vi "Autonomous Independent.vi"() -> ()   [LabVIEW 2016]
doc: "This VI is called when autonomous begins, and will automatically be terminated when autonomous ends. You can carry out timed or sensor driven robot movement independently without needing to return to the caller."
uses:
  <vilib>/Rock Robotics/WPI/Utilities/WPI_GetSetVariantRefNum.vi
  <vilib>/Rock Robotics/Network Tables/NT Read String.vi
  <vilib>/Rock Robotics/Network Tables/NT Write Numeric Array.vi
  <vilib>/Rock Robotics/WPI/RobotDrive/WPI_RobotDriveArcadeDrive_Standard(NoSaturation).vi
  <vilib>/Rock Robotics/Network Tables/NT Write Number.vi
  Robot Global Data.vi
  <vilib>/Rock Robotics/WPI/Counter/WPI_CounterDigitalInputToDigitalSource.vi
  <vilib>/Rock Robotics/SystemInterfaces/DIO/FPGA_DIOChannel.ctl
panel:
  out "Hook Center Cons":dbl
  out "gyro":dbl
  out "sonar distance (inches)":dbl
  out "Encoder Loop":dbl
  out "Encoder Loop":string
  out "Current Movement, for debugging 2":T1 {"Y Joystick Value" scale=1.0..-1.0; "X Joystick Value" scale=-1.0..1.0}
  in  "Array of robot movements 2":T2(array[cluster])=[{"X Joystick Value"=0.39393939393939403, "Y Joystick Value"=0.0, "Delay (sec)"=1.0, "Movement Name"="turn"}, {"X Joystick Value"=-0.3737373737373737, "Y Joystick Value"=0.0, "Delay (sec)"=1.0, "Movement Name"="turn back"}] {"Y Joystick Value" scale=1.0..-1.0; "X Joystick Value" scale=-1.0..1.0}
  out "Current Movement, for debugging":T1 {"Y Joystick Value" scale=1.0..-1.0; "X Joystick Value" scale=-1.0..1.0}
  in  "Array of robot movements":T2(array[cluster])=[{"X Joystick Value"=0.39393939393939403, "Y Joystick Value"=0.0, "Delay (sec)"=1.0, "Movement Name"="turn"}, {"X Joystick Value"=-0.3737373737373737, "Y Joystick Value"=0.0, "Delay (sec)"=1.0, "Movement Name"="turn back"}] {"Y Joystick Value" scale=1.0..-1.0; "X Joystick Value" scale=-1.0..1.0}
  # "Sensor Readings\nConstanly updated in\nwhile loopes"
  # "Be sure to right-click and choose Data Operations>>Make Current Value default if you want to save the array values with the VI"
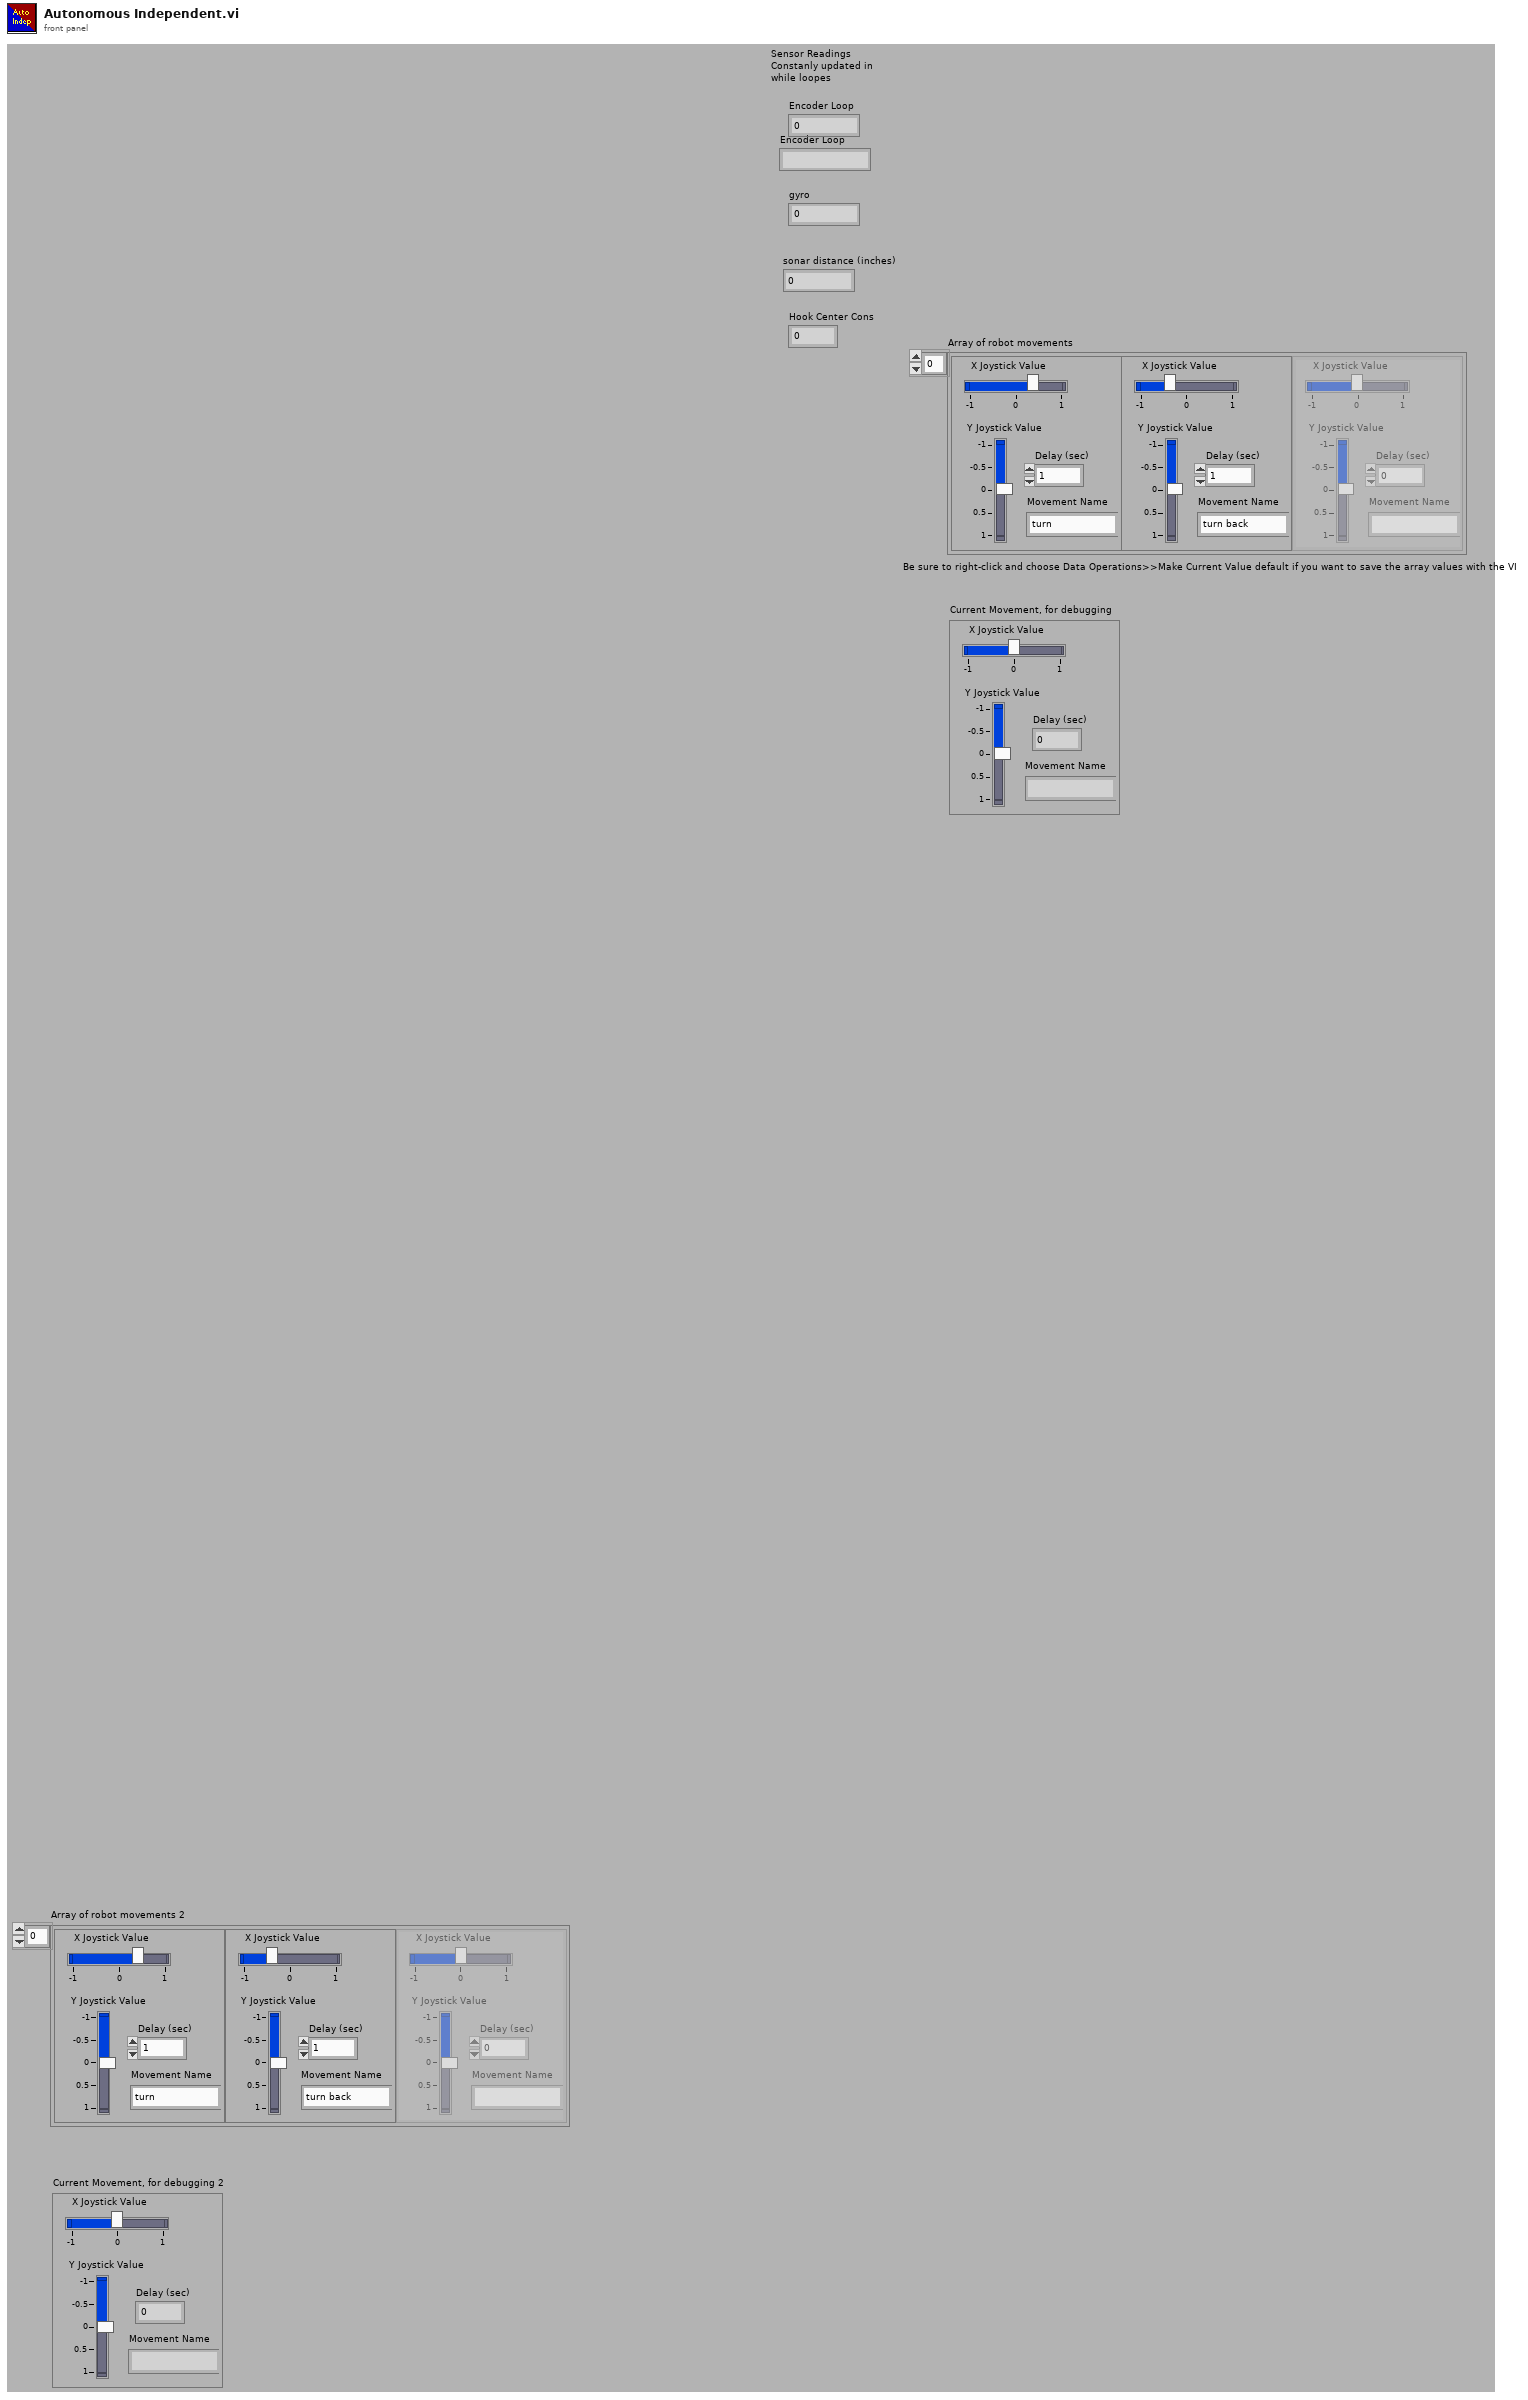
[diagram p1: front panel]
types:
  T1 = cluster{"X Joystick Value":dbl, "Y Joystick Value":dbl, "Delay (sec)":dbl, "Movement Name":string}
  T2 = cluster{"X Joystick Value":dbl, "Y Joystick Value":dbl, "Delay (sec)":dbl, "Movement Name":string}[]
  T3 = typedef "FPGA_DIOChannel.ctl" = enum8{"DIO 0", "DIO 1", "DIO 2", "DIO 3", "DIO 4", "DIO 5", "DIO 6", "DIO 7", "DIO 8", "DIO 9", "DIO MXP 0", "DIO MXP 1", "DIO MXP 2", "DIO MXP 3", "DIO MXP 4", "DIO MXP 5", "DIO MXP 6", "DIO MXP 7", "DIO MXP 8", "DIO MXP 9", "DIO MXP 10", "DIO MXP 11", "DIO MXP 12", "DIO MXP 13", "DIO MXP 14", "DIO MXP 15", "SPI Port CS1", "SPI Port CS2", "SPI Port CS3", "SPI Port MISO", "SPI Port MOSI", "Invalid"}
  T4 = typedef "WPI_DigitalInputDevRef.ctl" = cluster{"DevStatus":errorcluster, "DIO Channel":T3}
  T5 = typedef "FPGA_CounterEncoderSourceConvertionLVSourceType.ctl" = cluster{"DevStatus":errorcluster, "AnalogTriggerMode?":bool, "DigitalMode":cluster{"DIO Channel":T6}, "AnalogTriggerMode":cluster{"AnalogTriggerIndex":T7, "OutputType":T8}}
  T6 = typedef "FPGA_DIODigitalSourceChannel.ctl" = enum8{"DIO 0", "DIO 1", "DIO 2", "DIO 3", "DIO 4", "DIO 5", "DIO 6", "DIO 7", "DIO 8", "DIO 9", "DIO MXP 0", "DIO MXP 1", "DIO MXP 2", "DIO MXP 3", "DIO MXP 4", "DIO MXP 5", "DIO MXP 6", "DIO MXP 7", "DIO MXP 8", "DIO MXP 9", "DIO MXP 10", "DIO MXP 11", "DIO MXP 12", "DIO MXP 13", "DIO MXP 14", "DIO MXP 15", "Disabled"}
  T7 = typedef "FPGA_AnalogTriggerIndex.ctl" = enum8{"Trig 0", "Trig 1", "Trig 2", "Trig 3", "Trig 4", "Trig 5", "Trig 6", "Trig 7", "Invalid"}
  T8 = typedef "FPGA_AnalogTriggerOutType.ctl" = enum16{"InWindow", "TriggerState", "Rising", "Falling"}
  T9 = typedef "WPI_EncoderDevRef.ctl" = cluster{"DevStatus":errorcluster, "EncoderIndex":T10, "CounterIndex":T11, "DistancePerCount":dbl, "Decoding Type":T12}
  T10 = typedef "FPGA_EncoderIdx.ctl" = enum8{"Enc 0", "Enc 1", "Enc 2", "Enc 3", "Enc 4", "Enc 5", "Enc 6", "Enc 7", "Invalid"}
  T11 = typedef "FPGA_CounterCtrSystemIndex.ctl" = enum8{"Ctr 0", "Ctr 1", "Ctr 2", "Ctr 3", "Ctr 4", "Ctr 5", "Ctr 6", "Ctr 7", "Invalid"}
  T12 = typedef "WPI_EncoderType.ctl" = enum16{"1x", "2x", "4x"}
  T13 = typedef "WPI_JoystickDevRef.ctl" = cluster{"Device":T14}
  T14 = typedef "WPI_JoystickDeviceEnum.ctl" = enum16{"USB 0", "USB 1", "USB 2", "USB 3", "USB 4", "USB 5"}
  T15 = typedef "WPI_DriverStationPositionInfo.ctl" = enum16{"1", "2", "3"}
  T16 = typedef "WPI_RobotDriveDevRef.ctl" = cluster{"DevStatus":errorcluster, "Motors[]":T17[], "Square Inputs":bool, "Max Output":dbl}
  T17 = typedef "WPI_MotorControlDeviceRef.ctl" = cluster{"DeviceStatus":errorcluster, "Type":T18, "PWM":cluster{"PWM Channel":T19, "DeadBand":T20}, "CAN":cluster{"Device Number":u8, "SetOutput VI Ref":variant, "GetOutput VI Ref":variant, "Enable VI Ref":variant, "Disable VI Ref":variant, "Data":variant}, "Invert":bool}
  T18 = typedef "WPI_MotorControlType.ctl" = enum16{"PWM", "CAN"}
  T19 = typedef "FPGA_DIOPWMChannel.ctl" = enum8{"PWM 0", "PWM 1", "PWM 2", "PWM 3", "PWM 4", "PWM 5", "PWM 6", "PWM 7", "PWM 8", "PWM 9", "PWM MXP 0", "PWM MXP 1", "PWM MXP 2", "PWM MXP 3", "PWM MXP 4", "PWM MXP 5", "PWM MXP 6", "PWM MXP 7", "PWM MXP 8", "PWM MXP 9", "Invalid"}
  T20 = typedef "WPI_PWMDeadband.ctl" = cluster{"Name":string, "maxPositivePwm":i32, "minPositivePwm":i32, "centerPwm":i32, "maxNegativePwm":i32, "minNegativePwm":i32, "angularRange":u16}
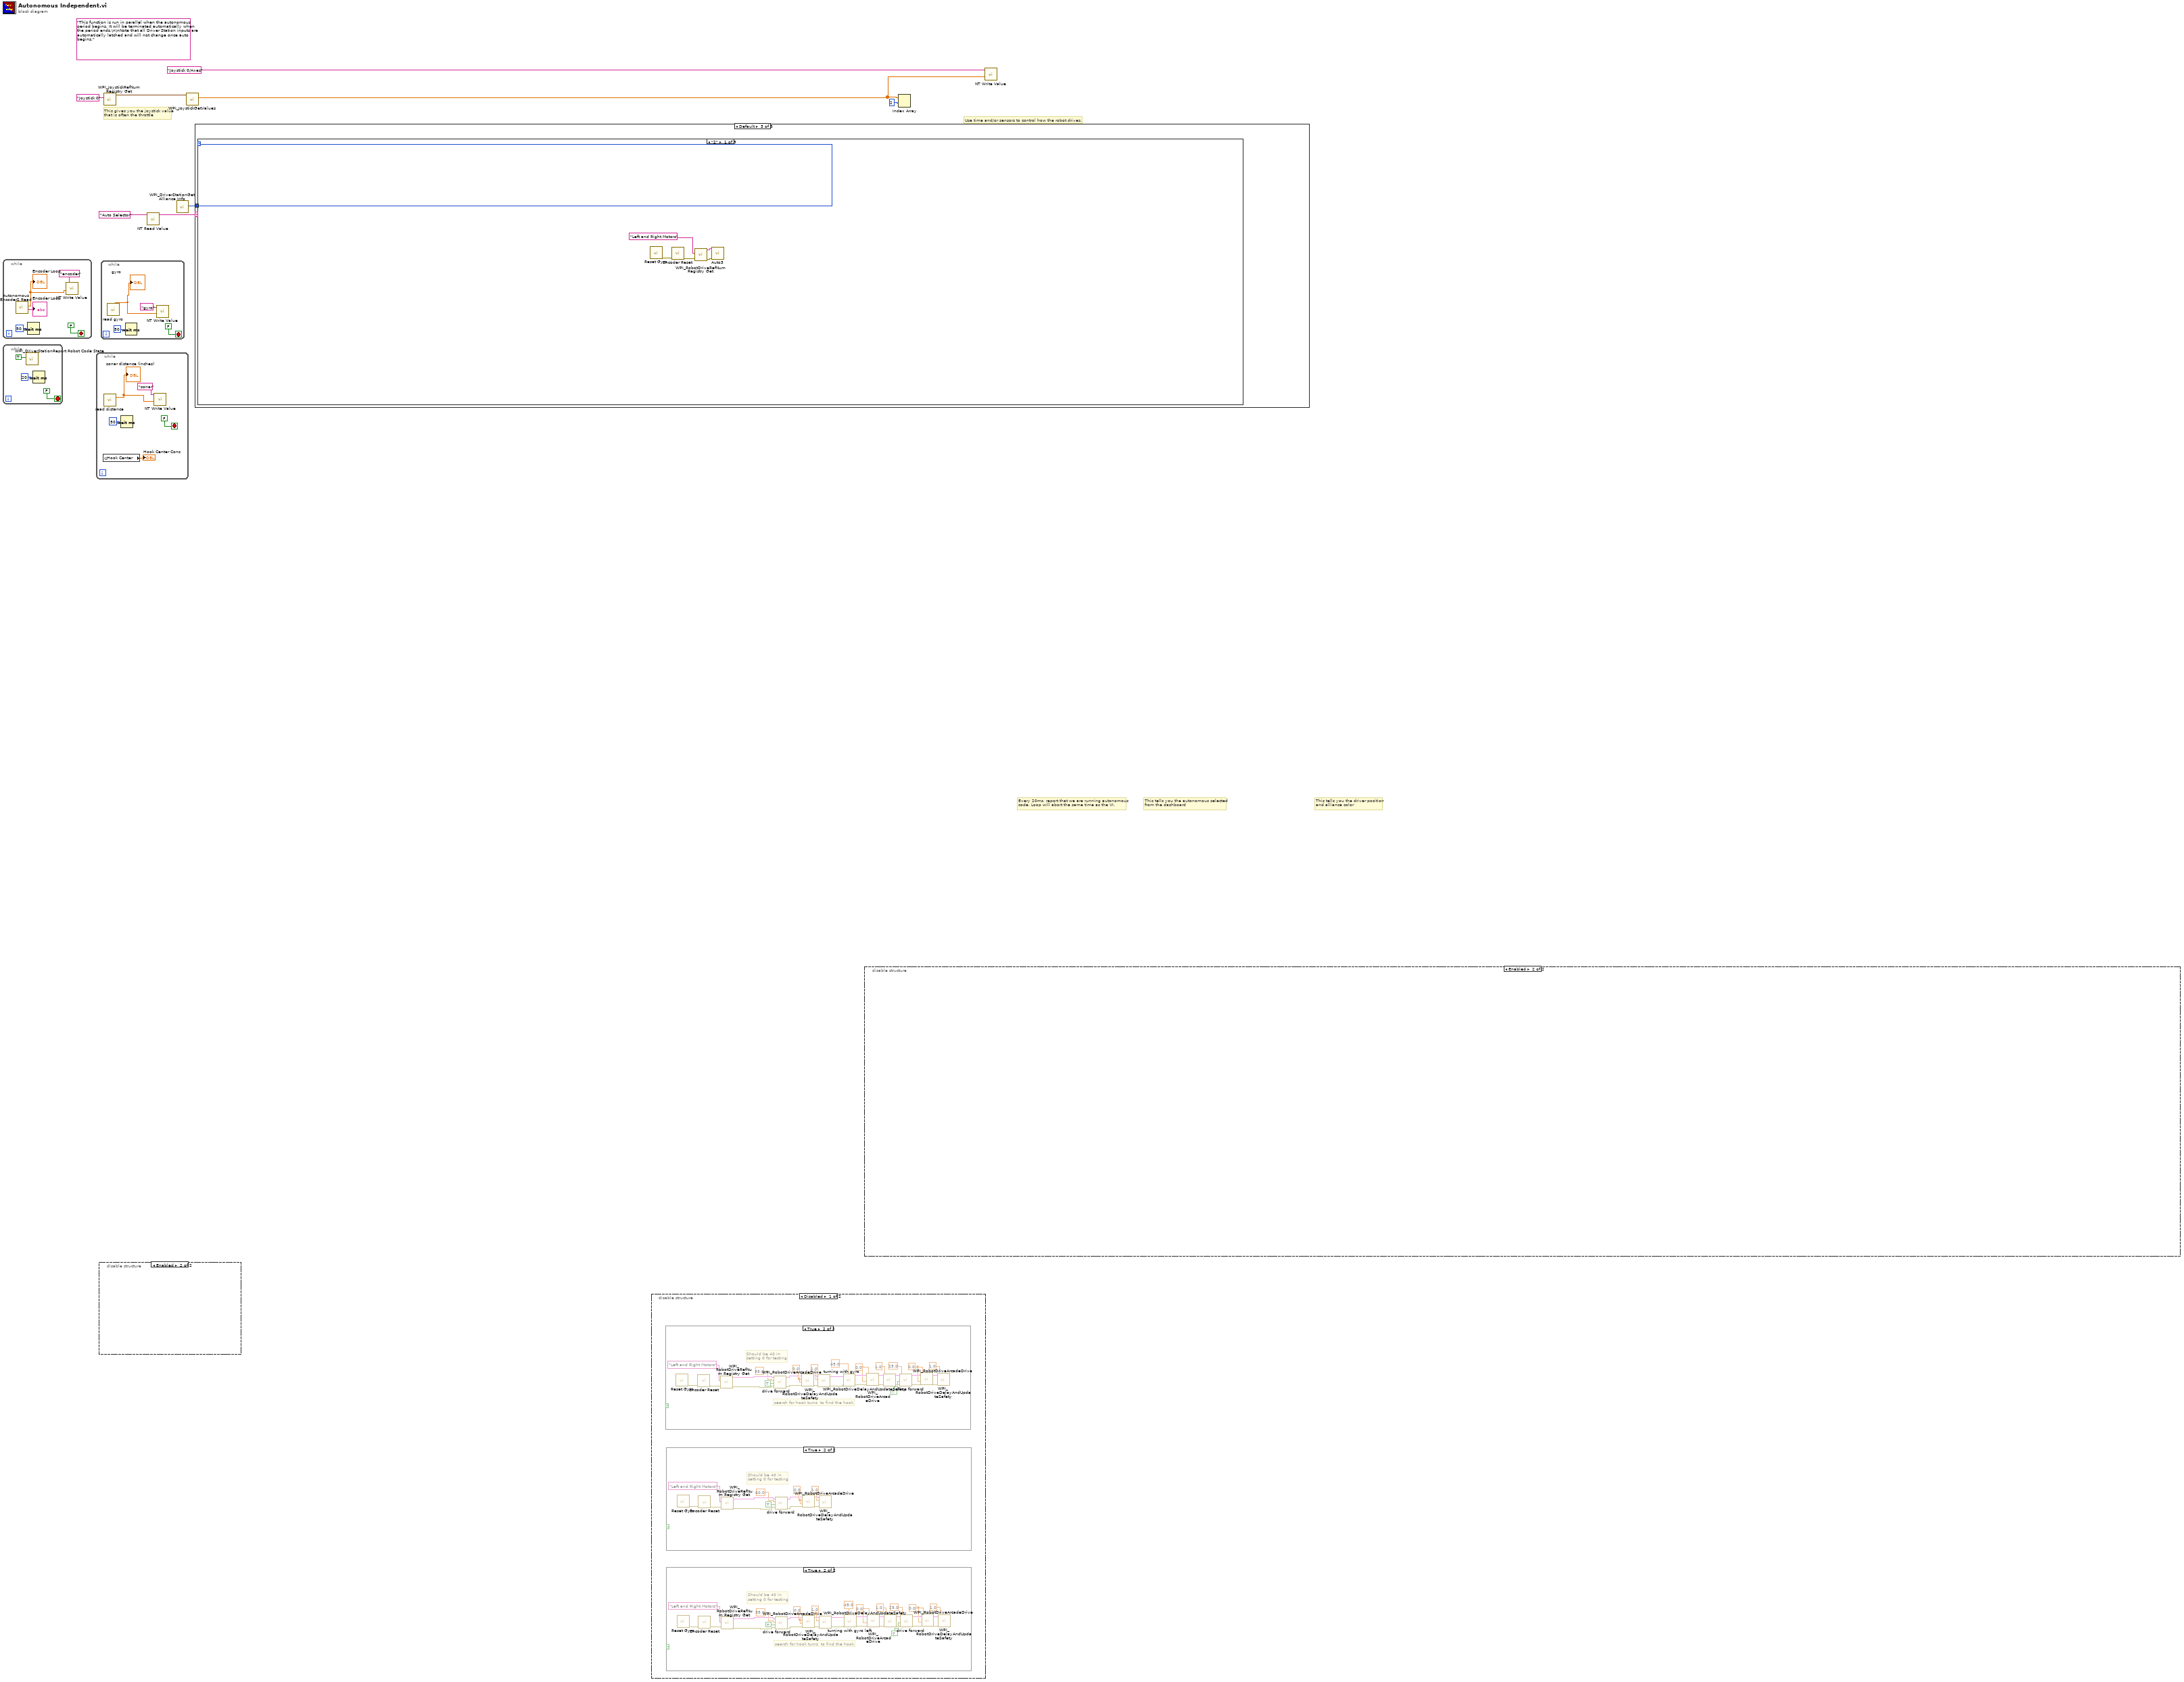
[diagram p0: block diagram]
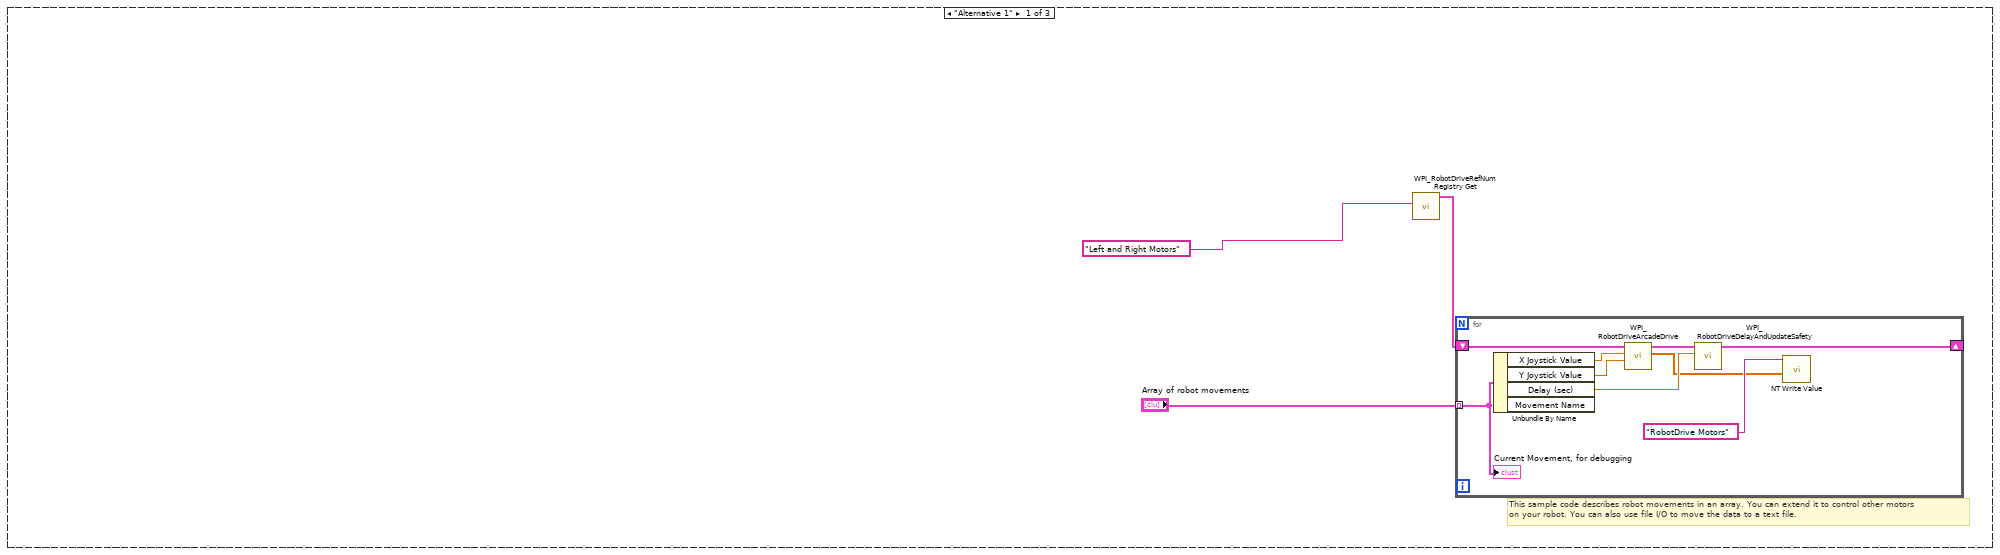
[diagram p6: hidden frame]
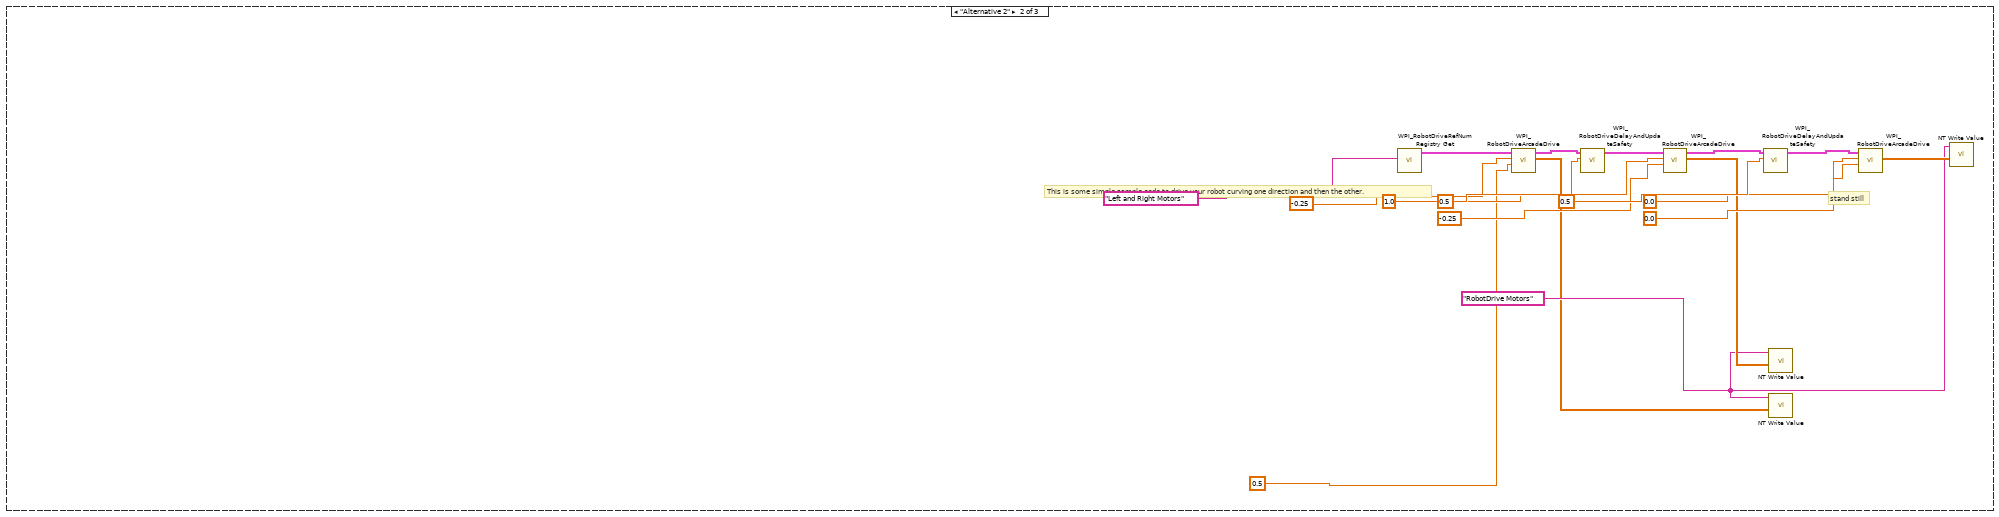
[diagram p7: hidden frame]
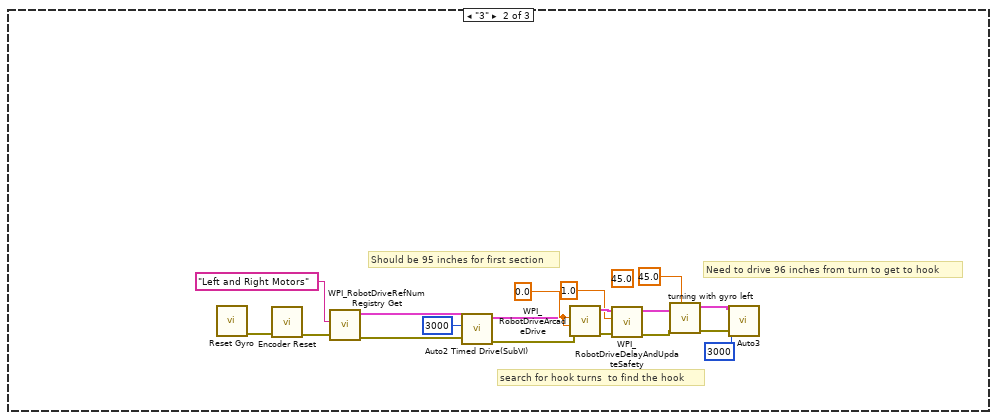
[diagram p8: hidden frame]
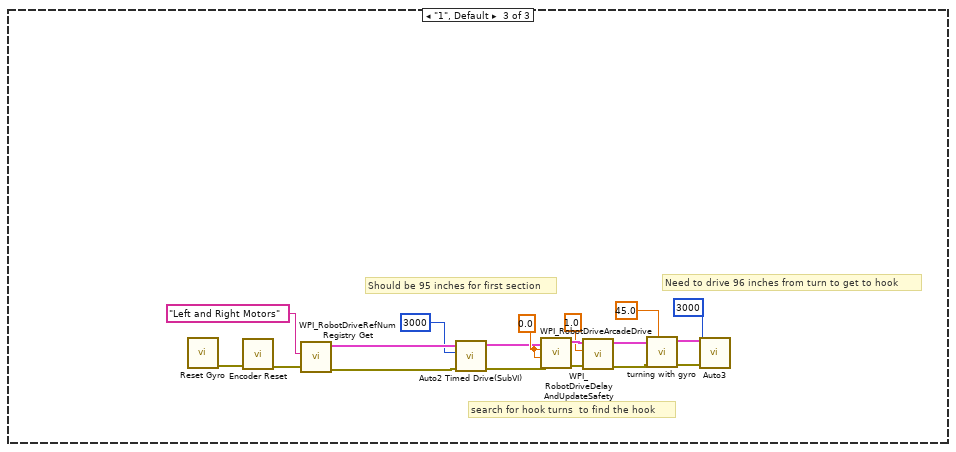
[diagram p9: hidden frame]
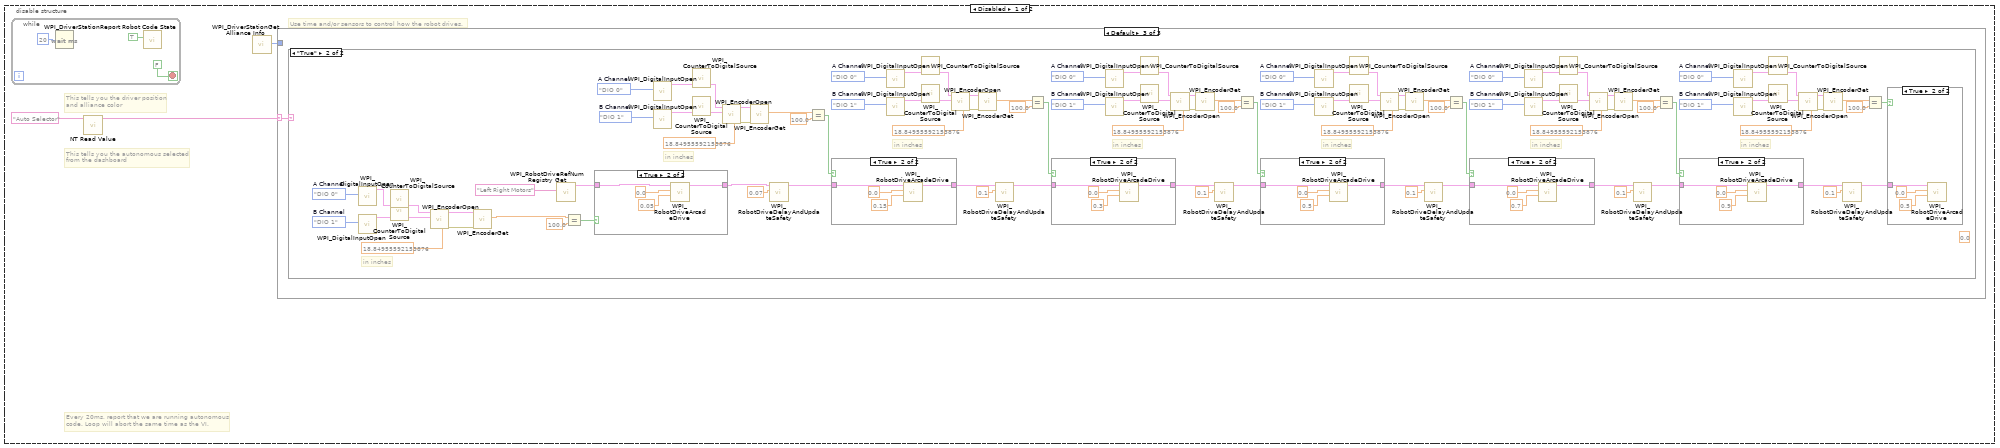
[diagram p10: hidden frame]
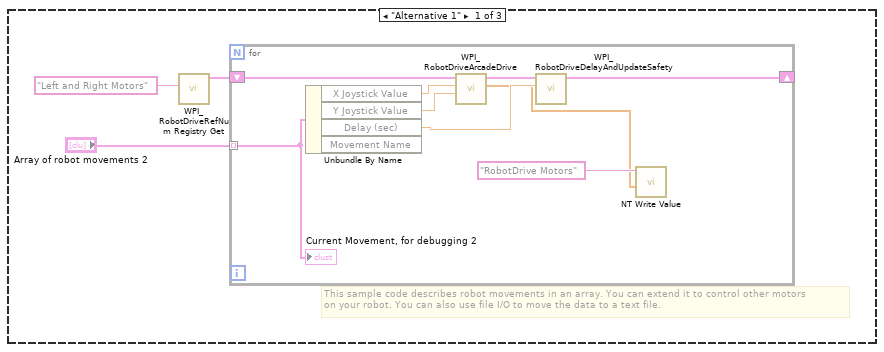
[diagram p11: hidden frame]
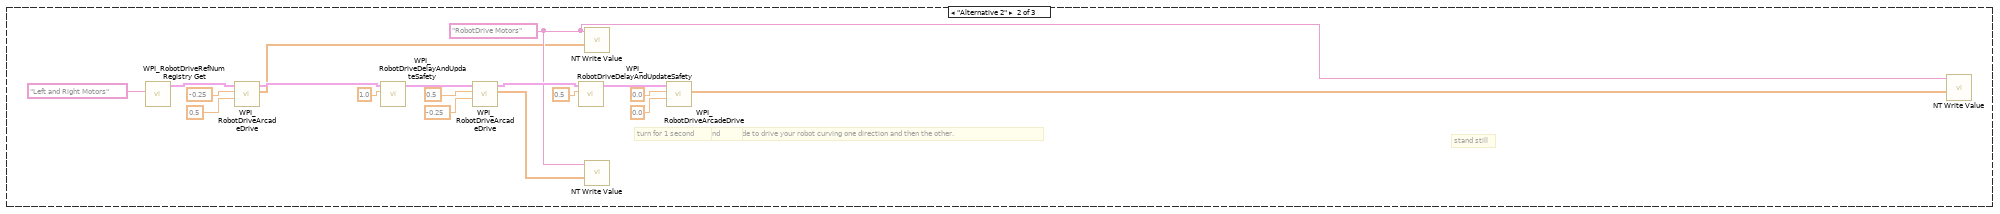
[diagram p12: hidden frame]
diagram:
  (unwired) "This function is run in parallel when the autonomous period begins. It will be terminated automatically when the period ends.\n\nNote that all Driver Station inputs are automatically latched and will not change once auto begins."
  # "This tells you the autonomous selected\nfrom the dashboard"
  # "Every 20ms, report that we are running autonomous\ncode. Loop will abort the same time as the VI."
  # "This gives you the joystick value\nthat is often the throttle"
  # "Use time and/or sensors to control how the robot drives."
  # "This tells you the driver position\nand alliance color"
  n1 = while {
    stop <- FALSE stop-if-true
    n2 = call "Autonomous Encoder2 Read.vi"() -> ("Encoder Direction"=→"Encoder Loop":string, "Encoder Distance"=w10:dbl)  [unwired: 9 in, 1 out]
    "Encoder Loop" <- w10
    n3 = Wait (ms)(milliseconds to wait=u32 50) -> ()  [unwired: 1 out]
    n4 = call-poly <vilib>:"NT Write Value.vi"("Numeric"=w10, "Name"="encoder") -> ()  [unwired: 9 in, 1 out]
  }
  n5 = while {
    stop <- FALSE stop-if-true
    n6 = call <vilib>:"WPI_DriverStationReport Robot Code State.vi"("Autonomous"=TRUE) -> ()  [unwired: 10 in, 1 out]
    n7 = Wait (ms)(milliseconds to wait=u32 20) -> ()  [unwired: 1 out]
  }
  n8 = while {
    stop <- FALSE stop-if-true
    n9 = global read "Robot Global Data.vi" "Hook Center"() -> (→"Hook Center Cons":dbl)
    n10 = call "read distance.vi"() -> ("Distance 2"=w19:dbl)  [unwired: 10 in, 1 out]
    "sonar distance (inches)" <- w19
    n11 = Wait (ms)(milliseconds to wait=u32 50) -> ()  [unwired: 1 out]
    n12 = call-poly <vilib>:"NT Write Value.vi"("Numeric"=w19, "Name"="sonar") -> ()  [unwired: 9 in, 1 out]
  }
  n13 = disable-structure shown="Enabled" {
    frame Disabled {
      w35 = FPGA_DIOChannel."DIO 1"  # B Channel
      w34 = FPGA_DIOChannel."DIO 0"  # A Channel
      # "in inches"
      n14 = call <vilib>:"WPI_DigitalInputOpen.vi"("DIO Channel"=w34) -> ("DigitalInputDevRef"=w31:T4)  [unwired: 1 in, 9 out]
      n15 = call <vilib>:"WPI_DigitalInputOpen.vi"("DIO Channel"=w35) -> ("DigitalInputDevRef"=w32:T4)  [unwired: 1 in, 9 out]
      n16 = call-poly <vilib>:"WPI_CounterToDigitalSource.vi"("DigitalInputDevRef"=w31) -> ("Digital Source"=w30:T5)  [unwired: 6 out]
      n17 = call-poly <vilib>:"WPI_CounterToDigitalSource.vi"("DigitalInputDevRef"=w32) -> ("Digital Source"=w33:T5)  [unwired: 6 out]
      n18 = call <vilib>:"WPI_EncoderOpen.vi"("DistancePerCount"=18.84955592153876, "Invert Direction (False)"=FALSE, "BSource"=w33, "ASource"=w30) -> ("error out"=w28:errorcluster, "EncoderDevRef"=w29:T9)  [unwired: 4 in, 2 out]
      n19 = call-poly <vilib>:"NT Write Value.vi"("Name"="Encoder Distance") -> ()  [unwired: 10 in, 1 out]
      n20 = call <vilib>:"WPI_EncoderRefNum Registry Set.vi"("error in (no error)"=w28, "refnum name"="Encoder", "EncoderDevRef"=w29) -> ("error out"=w26:errorcluster, "EncoderDevRef"=w27:T9)  [unwired: 7 in]
      n21 = call <vilib>:"WPI_EncoderGet.vi"("error in (no error)"=w26, "EncoderDevRef"=w27) -> ()  [unwired: 4 in, 6 out]
    }
    frame Enabled {
    }
  }
  n22 = while {
    stop <- FALSE stop-if-true
    n23 = call "read gyro.vi"() -> ("Angle 2"=w37:dbl)  [unwired: 10 in, 1 out]
    "gyro" <- w37
    n24 = Wait (ms)(milliseconds to wait=u32 50) -> ()  [unwired: 1 out]
    n25 = call-poly <vilib>:"NT Write Value.vi"("Numeric"=w37, "Name"="gyro") -> ()  [unwired: 9 in, 1 out]
  }
  n26 = call <vilib>:"WPI_JoystickRefNum Registry Get.vi"("refnum name"="Joystick 0") -> ("JoystickDevRef"=w7:T13)  [unwired: 1 in, 9 out]
  n27 = call-poly <vilib>:"NT Read Value.vi"("Name"="Auto Selector") -> ("String"=w4:string)  [unwired: 9 in, 1 out]
  n28 = call <vilib>:"WPI_DriverStationGet Alliance Info.vi"() -> ("Position"=w1:T15)  [unwired: 11 out]
  n29 = call <vilib>:"WPI_JoystickGetValues.vi"("JoystickDevRef"=w7) -> ("Axes"=w3:dbl[])  [unwired: 6 in, 4 out]
  n30 = case shown="Default" w4 {
    tunnel: w1 -> [_ _ w70]
    frame "Alternative 1" {
      # "This sample code describes robot movements in an array. You can extend it to control other motors\non your robot. You can also use file I/O to move the data to a text file."
      n31 = call <vilib>:"WPI_RobotDriveRefNum Registry Get.vi"("refnum name"="Left and Right Motors") -> ("RobotDriveDevRef"=w41:T16)  [unwired: 1 in, 9 out]
      n32 = for {
        shift-right: [w49] -> _
        shift-left: w41 -> [w50]
        tunnel: "Array of robot movements" -> [w45] mode=indexing
        n33 = Unbundle By Name(w45) -> ("X Joystick Value"=w48:dbl, "Y Joystick Value"=w47:dbl, "Delay (sec)"=w46:dbl)  [unwired: 1 out]
        n34 = call-poly <vilib>:"WPI_RobotDriveArcadeDrive.vi"("Y axis value"=w47, "X axis value"=w48, "RobotDriveDevRef"=w50) -> ("Motor Values"=w43:dbl[], "RobotDriveDevRef"=w51:T16)  [unwired: 1 in, 6 out]
        n35 = call <vilib>:"WPI_RobotDriveDelayAndUpdateSafety.vi"("Delay (s)"=w46, "RobotDriveDevRef"=w51) -> ("RobotDriveDevRef 2"=w49:T16)  [unwired: 8 in, 1 out]
        n36 = call-poly <vilib>:"NT Write Value.vi"("Numeric Array"=w43, "Name"="RobotDrive Motors") -> ()  [unwired: 9 in, 1 out]
        "Current Movement, for debugging" <- w45
      }
    }
    frame "Alternative 2" {
      w53 = "RobotDrive Motors" ("Name")
      # "This is some simple sample code to drive your robot curving one direction and then the other."
      # "stand still"
      n37 = call <vilib>:"WPI_RobotDriveRefNum Registry Get.vi"("refnum name"="Left and Right Motors") -> ("RobotDriveDevRef"=w69:T16)  [unwired: 1 in, 9 out]
      n38 = call-poly <vilib>:"WPI_RobotDriveArcadeDrive.vi"("Y axis value"=0.5 ("X axis value"), "X axis value"=-0.25, "RobotDriveDevRef"=w69) -> ("Motor Values"=w52:dbl[], "RobotDriveDevRef"=w62:T16)  [unwired: 1 in, 6 out]
      n39 = call <vilib>:"WPI_RobotDriveDelayAndUpdateSafety.vi"("Delay (s)"=1.0, "RobotDriveDevRef"=w62) -> ("RobotDriveDevRef 2"=w63:T16)  [unwired: 8 in, 1 out]
      n40 = call-poly <vilib>:"WPI_RobotDriveArcadeDrive.vi"("Y axis value"=-0.25 ("X axis value"), "X axis value"=0.5, "RobotDriveDevRef"=w63) -> ("Motor Values"=w54:dbl[], "RobotDriveDevRef"=w64:T16)  [unwired: 1 in, 6 out]
      n41 = call <vilib>:"WPI_RobotDriveDelayAndUpdateSafety.vi"("Delay (s)"=0.5, "RobotDriveDevRef"=w64) -> ("RobotDriveDevRef 2"=w65:T16)  [unwired: 8 in, 1 out]
      n42 = call-poly <vilib>:"NT Write Value.vi"("Numeric Array"=w54, "Name"=w53) -> ()  [unwired: 9 in, 1 out]
      n43 = call-poly <vilib>:"NT Write Value.vi"("Numeric Array"=w52, "Name"=w53) -> ()  [unwired: 9 in, 1 out]
      n44 = call-poly <vilib>:"WPI_RobotDriveArcadeDrive.vi"("Y axis value"=0.0 ("X axis value"), "X axis value"=0.0, "RobotDriveDevRef"=w65) -> ("Motor Values"=w55:dbl[])  [unwired: 1 in, 7 out]
      n45 = call-poly <vilib>:"NT Write Value.vi"("Numeric Array"=w55, "Name"=w53) -> ()  [unwired: 9 in, 1 out]
    }
    frame Default {
      n46 = case shown="\"2\"" w70 {
        frame "2" {
          n47 = call "Reset Gyro.vi"() -> ("error out"=w73:errorcluster)  [unwired: 11 in]
          n48 = call "Encoder Reset.vi"("error in (no error)"=w73) -> ("error out"=w74:errorcluster)  [unwired: 10 in]
          n49 = call <vilib>:"WPI_RobotDriveRefNum Registry Get.vi"("error in (no error)"=w74, "refnum name"="Left and Right Motors") -> ("error out"=w71:errorcluster, "RobotDriveDevRef"=w72:T16)  [unwired: 8 out]
          n50 = call "Auto3.vi"("RobotDriveDevRef"=w72, "error in (no error)"=w71) -> ()  [unwired: 6 in, 8 out]
        }
        frame "3" {
          (unwired) 45.0 ("desired angle")
          w87 = 0.0 ("X axis value")
          # "Should be 95 inches for first section"
          # "Need to drive 96 inches from turn to get to hook"
          # "search for hook turns  to find the hook"
          n51 = call "Reset Gyro.vi"() -> ("error out"=w91:errorcluster)  [unwired: 11 in]
          n52 = call "Encoder Reset.vi"("error in (no error)"=w91) -> ("error out"=w92:errorcluster)  [unwired: 10 in]
          n53 = call <vilib>:"WPI_RobotDriveRefNum Registry Get.vi"("error in (no error)"=w92, "refnum name"="Left and Right Motors") -> ("error out"=w85:errorcluster, "RobotDriveDevRef"=w86:T16)  [unwired: 8 out]
          n54 = call "Auto2 Timed Drive(SubVI).vi"("error in (no error)"=w85, "milliseconds to wait"=u32 3000, "RobotDriveDevRef in"=w86) -> ("error out"=w83:errorcluster, "RobotDriveDevRef out"=w84:T16)  [unwired: 7 in]
          n55 = call-poly <vilib>:"WPI_RobotDriveArcadeDrive.vi"("error in (no error)"=w83, "Y axis value"=w87, "X axis value"=w87, "RobotDriveDevRef"=w84) -> ("error out"=w89:errorcluster, "RobotDriveDevRef"=w90:T16)  [unwired: 6 out]
          n56 = call <vilib>:"WPI_RobotDriveDelayAndUpdateSafety.vi"("error in (no error)"=w89, "Delay (s)"=1.0, "RobotDriveDevRef"=w90) -> ("error out"=w79:errorcluster, "RobotDriveDevRef 2"=w80:T16)  [unwired: 7 in]
          n57 = call "turning with gyro left.vi"("desired angle"=45.0, "error in (no error)"=w79, "RobotDriveDevRef"=w80) -> ("error out"=w77:errorcluster, "RobotDriveDevRef 2"=w78:T16)  [unwired: 6 in, 1 out]
          n58 = call "Auto3.vi"("RobotDriveDevRef"=w78, "milliseconds to wait"=u32 3000, "error in (no error)"=w77) -> ()  [unwired: 5 in, 8 out]
        }
        frame "1", Default {
          w105 = 0.0 ("X axis value")
          # "Need to drive 96 inches from turn to get to hook"
          # "search for hook turns  to find the hook"
          # "Should be 95 inches for first section"
          n59 = call "Reset Gyro.vi"() -> ("error out"=w109:errorcluster)  [unwired: 11 in]
          n60 = call "Encoder Reset.vi"("error in (no error)"=w109) -> ("error out"=w110:errorcluster)  [unwired: 10 in]
          n61 = call <vilib>:"WPI_RobotDriveRefNum Registry Get.vi"("error in (no error)"=w110, "refnum name"="Left and Right Motors") -> ("error out"=w98:errorcluster, "RobotDriveDevRef"=w99:T16)  [unwired: 8 out]
          n62 = call "Auto2 Timed Drive(SubVI).vi"("error in (no error)"=w98, "milliseconds to wait"=u32 3000, "RobotDriveDevRef in"=w99) -> ("error out"=w96:errorcluster, "RobotDriveDevRef out"=w97:T16)  [unwired: 7 in]
          n63 = call-poly <vilib>:"WPI_RobotDriveArcadeDrive.vi"("error in (no error)"=w96, "Y axis value"=w105, "X axis value"=w105, "RobotDriveDevRef"=w97) -> ("error out"=w107:errorcluster, "RobotDriveDevRef"=w108:T16)  [unwired: 6 out]
          n64 = call <vilib>:"WPI_RobotDriveDelayAndUpdateSafety.vi"("error in (no error)"=w107, "Delay (s)"=1.0, "RobotDriveDevRef"=w108) -> ("error out"=w103:errorcluster, "RobotDriveDevRef 2"=w104:T16)  [unwired: 7 in]
          n65 = call "turning with gyro.vi"("desired angle"=45.0, "error in (no error)"=w103, "RobotDriveDevRef"=w104) -> ("error out"=w100:errorcluster, "RobotDriveDevRef 2"=w101:T16)  [unwired: 7 in]
          n66 = call "Auto3.vi"("RobotDriveDevRef"=w101, "milliseconds to wait"=u32 3000, "error in (no error)"=w100) -> ()  [unwired: 5 in, 8 out]
        }
      }
    }
  }
  n67 = disable-structure shown="Disabled" {
    frame Disabled {
      n68 = case shown="True" {
        selector: _ -> [_ _]
        frame False {
        }
        frame True {
          w160 = 0.0 ("X axis value")
          w171 = 0.0 ("X axis value")
          w178 = 0.0 ("X axis value")
          # "search for hook turns  to find the hook"
          # "Should be 40 in\nsetting 0 for testing"
          n69 = call "Reset Gyro.vi"() -> ("error out"=w185:errorcluster)  [unwired: 11 in]
          n70 = call "Encoder Reset.vi"("error in (no error)"=w185) -> ("error out"=w187:errorcluster)  [unwired: 10 in]
          n71 = call <vilib>:"WPI_RobotDriveRefNum Registry Get.vi"("error in (no error)"=w187, "refnum name"="Left and Right Motors") -> ("error out"=w184:errorcluster, "RobotDriveDevRef"=w186:T16)  [unwired: 8 out]
          n72 = call "drive forward.vi"("error in (no error)"=w184, "forward"=TRUE, "desired distance"=95.0, "RobotDriveDevRef in"=w186) -> ("error out"=w176:errorcluster, "RobotDriveDevRef out"=w177:T16)  [unwired: 6 in]
          n73 = call-poly <vilib>:"WPI_RobotDriveArcadeDrive.vi"("error in (no error)"=w176, "Y axis value"=w178, "X axis value"=w178, "RobotDriveDevRef"=w177) -> ("error out"=w180:errorcluster, "RobotDriveDevRef"=w181:T16)  [unwired: 6 out]
          n74 = call <vilib>:"WPI_RobotDriveDelayAndUpdateSafety.vi"("error in (no error)"=w180, "Delay (s)"=1.0, "RobotDriveDevRef"=w181) -> ("error out"=w174:errorcluster, "RobotDriveDevRef 2"=w175:T16)  [unwired: 7 in]
          n75 = call "turning with gyro.vi"("desired angle"=45.0, "error in (no error)"=w174, "RobotDriveDevRef"=w175) -> ("error out"=w168:errorcluster, "RobotDriveDevRef 2"=w172:T16)  [unwired: 7 in]
          n76 = call-poly <vilib>:"WPI_RobotDriveArcadeDrive.vi"("error in (no error)"=w168, "Y axis value"=w171, "X axis value"=w171, "RobotDriveDevRef"=w172) -> ("error out"=w169:errorcluster, "RobotDriveDevRef"=w170:T16)  [unwired: 6 out]
          n77 = call <vilib>:"WPI_RobotDriveDelayAndUpdateSafety.vi"("error in (no error)"=w169, "Delay (s)"=1.0, "RobotDriveDevRef"=w170) -> ("error out"=w166:errorcluster, "RobotDriveDevRef 2"=w165:T16)  [unwired: 7 in]
          n78 = call "drive forward.vi"("error in (no error)"=w166, "forward"=TRUE, "desired distance"=25.0, "RobotDriveDevRef in"=w165) -> ("error out"=w161:errorcluster, "RobotDriveDevRef out"=w162:T16)  [unwired: 6 in]
          n79 = call-poly <vilib>:"WPI_RobotDriveArcadeDrive.vi"("error in (no error)"=w161, "Y axis value"=w160, "X axis value"=w160, "RobotDriveDevRef"=w162) -> ("error out"=w158:errorcluster, "RobotDriveDevRef"=w159:T16)  [unwired: 6 out]
          n80 = call <vilib>:"WPI_RobotDriveDelayAndUpdateSafety.vi"("error in (no error)"=w158, "Delay (s)"=1.0, "RobotDriveDevRef"=w159) -> ()  [unwired: 7 in, 2 out]
        }
      }
      n81 = case shown="True" {
        selector: _ -> [_ _]
        frame False {
        }
        frame True {
          w146 = 0.0 ("X axis value")
          # "Should be 40 in\nsetting 0 for testing"
          n82 = call "Reset Gyro.vi"() -> ("error out"=w153:errorcluster)  [unwired: 11 in]
          n83 = call "Encoder Reset.vi"("error in (no error)"=w153) -> ("error out"=w155:errorcluster)  [unwired: 10 in]
          n84 = call <vilib>:"WPI_RobotDriveRefNum Registry Get.vi"("error in (no error)"=w155, "refnum name"="Left and Right Motors") -> ("error out"=w152:errorcluster, "RobotDriveDevRef"=w154:T16)  [unwired: 8 out]
          n85 = call "drive forward.vi"("error in (no error)"=w152, "forward"=TRUE, "desired distance"=60.0, "RobotDriveDevRef in"=w154) -> ("error out"=w144:errorcluster, "RobotDriveDevRef out"=w145:T16)  [unwired: 6 in]
          n86 = call-poly <vilib>:"WPI_RobotDriveArcadeDrive.vi"("error in (no error)"=w144, "Y axis value"=w146, "X axis value"=w146, "RobotDriveDevRef"=w145) -> ("error out"=w148:errorcluster, "RobotDriveDevRef"=w149:T16)  [unwired: 6 out]
          n87 = call <vilib>:"WPI_RobotDriveDelayAndUpdateSafety.vi"("error in (no error)"=w148, "Delay (s)"=1.0, "RobotDriveDevRef"=w149) -> ()  [unwired: 7 in, 2 out]
        }
      }
      n88 = case shown="True" {
        selector: _ -> [_ _]
        frame False {
        }
        frame True {
          w115 = 0.0 ("X axis value")
          w126 = 0.0 ("X axis value")
          w133 = 0.0 ("X axis value")
          # "search for hook turns  to find the hook"
          # "Should be 40 in\nsetting 0 for testing"
          n89 = call "Reset Gyro.vi"() -> ("error out"=w140:errorcluster)  [unwired: 11 in]
          n90 = call "Encoder Reset.vi"("error in (no error)"=w140) -> ("error out"=w142:errorcluster)  [unwired: 10 in]
          n91 = call <vilib>:"WPI_RobotDriveRefNum Registry Get.vi"("error in (no error)"=w142, "refnum name"="Left and Right Motors") -> ("error out"=w139:errorcluster, "RobotDriveDevRef"=w141:T16)  [unwired: 8 out]
          n92 = call "drive forward.vi"("error in (no error)"=w139, "forward"=TRUE, "desired distance"=95.0, "RobotDriveDevRef in"=w141) -> ("error out"=w131:errorcluster, "RobotDriveDevRef out"=w132:T16)  [unwired: 6 in]
          n93 = call-poly <vilib>:"WPI_RobotDriveArcadeDrive.vi"("error in (no error)"=w131, "Y axis value"=w133, "X axis value"=w133, "RobotDriveDevRef"=w132) -> ("error out"=w135:errorcluster, "RobotDriveDevRef"=w136:T16)  [unwired: 6 out]
          n94 = call <vilib>:"WPI_RobotDriveDelayAndUpdateSafety.vi"("error in (no error)"=w135, "Delay (s)"=1.0, "RobotDriveDevRef"=w136) -> ("error out"=w129:errorcluster, "RobotDriveDevRef 2"=w130:T16)  [unwired: 7 in]
          n95 = call "turning with gyro left.vi"("desired angle"=45.0, "error in (no error)"=w129, "RobotDriveDevRef"=w130) -> ("error out"=w123:errorcluster, "RobotDriveDevRef 2"=w127:T16)  [unwired: 6 in, 1 out]
          n96 = call-poly <vilib>:"WPI_RobotDriveArcadeDrive.vi"("error in (no error)"=w123, "Y axis value"=w126, "X axis value"=w126, "RobotDriveDevRef"=w127) -> ("error out"=w124:errorcluster, "RobotDriveDevRef"=w125:T16)  [unwired: 6 out]
          n97 = call <vilib>:"WPI_RobotDriveDelayAndUpdateSafety.vi"("error in (no error)"=w124, "Delay (s)"=1.0, "RobotDriveDevRef"=w125) -> ("error out"=w121:errorcluster, "RobotDriveDevRef 2"=w120:T16)  [unwired: 7 in]
          n98 = call "drive forward.vi"("error in (no error)"=w121, "forward"=TRUE, "desired distance"=25.0, "RobotDriveDevRef in"=w120) -> ("error out"=w116:errorcluster, "RobotDriveDevRef out"=w117:T16)  [unwired: 6 in]
          n99 = call-poly <vilib>:"WPI_RobotDriveArcadeDrive.vi"("error in (no error)"=w116, "Y axis value"=w115, "X axis value"=w115, "RobotDriveDevRef"=w117) -> ("error out"=w113:errorcluster, "RobotDriveDevRef"=w114:T16)  [unwired: 6 out]
          n100 = call <vilib>:"WPI_RobotDriveDelayAndUpdateSafety.vi"("error in (no error)"=w113, "Delay (s)"=1.0, "RobotDriveDevRef"=w114) -> ()  [unwired: 7 in, 2 out]
        }
      }
    }
    frame Enabled {
    }
  }
  n101 = disable-structure shown="Enabled" {
    frame Disabled {
      # "This tells you the autonomous selected\nfrom the dashboard"
      # "Every 20ms, report that we are running autonomous\ncode. Loop will abort the same time as the VI."
      # "Use time and/or sensors to control how the robot drives."
      # "This tells you the driver position\nand alliance color"
      n102 = while {
        stop <- FALSE stop-if-true
        n103 = Wait (ms)(milliseconds to wait=u32 20) -> ()  [unwired: 1 out]
        n104 = call <vilib>:"WPI_DriverStationReport Robot Code State.vi"("Autonomous"=TRUE) -> ()  [unwired: 10 in, 1 out]
      }
      n105 = call-poly <vilib>:"NT Read Value.vi"("Name"="Auto Selector") -> ("String"=w191:string)  [unwired: 9 in, 1 out]
      n106 = call <vilib>:"WPI_DriverStationGet Alliance Info.vi"() -> ("Position"=w190:T15)  [unwired: 11 out]
      n107 = case shown="Default" w191 {
        selector: w191 -> [_ _ w222]
        tunnel: w190 -> [_ _ _]
        frame "Alternative 1" {
          # "This sample code describes robot movements in an array. You can extend it to control other motors\non your robot. You can also use file I/O to move the data to a text file."
          n108 = call <vilib>:"WPI_RobotDriveRefNum Registry Get.vi"("refnum name"="Left and Right Motors") -> ("RobotDriveDevRef"=w193:T16)  [unwired: 1 in, 9 out]
          n109 = for {
            shift-right: [w201] -> _
            shift-left: w193 -> [w202]
            tunnel: "Array of robot movements 2" -> [w197] mode=indexing
            n110 = Unbundle By Name(w197) -> ("X Joystick Value"=w200:dbl, "Y Joystick Value"=w199:dbl, "Delay (sec)"=w198:dbl)  [unwired: 1 out]
            n111 = call-poly <vilib>:"WPI_RobotDriveArcadeDrive.vi"("Y axis value"=w199, "X axis value"=w200, "RobotDriveDevRef"=w202) -> ("Motor Values"=w195:dbl[], "RobotDriveDevRef"=w203:T16)  [unwired: 1 in, 6 out]
            n112 = call <vilib>:"WPI_RobotDriveDelayAndUpdateSafety.vi"("Delay (s)"=w198, "RobotDriveDevRef"=w203) -> ("RobotDriveDevRef 2"=w201:T16)  [unwired: 8 in, 1 out]
            n113 = call-poly <vilib>:"NT Write Value.vi"("Numeric Array"=w195, "Name"="RobotDrive Motors") -> ()  [unwired: 9 in, 1 out]
            "Current Movement, for debugging 2" <- w197
          }
        }
        frame "Alternative 2" {
          w205 = "RobotDrive Motors" ("Name")
          # "This is some simple sample code to drive your robot curving one direction and then the other."
          # "stand still"
          # "other way for 0.5 second"
          # "turn for 1 second"
          n114 = call <vilib>:"WPI_RobotDriveRefNum Registry Get.vi"("refnum name"="Left and Right Motors") -> ("RobotDriveDevRef"=w221:T16)  [unwired: 1 in, 9 out]
          n115 = call-poly <vilib>:"WPI_RobotDriveArcadeDrive.vi"("Y axis value"=0.5 ("X axis value"), "X axis value"=-0.25, "RobotDriveDevRef"=w221) -> ("Motor Values"=w204:dbl[], "RobotDriveDevRef"=w214:T16)  [unwired: 1 in, 6 out]
          n116 = call <vilib>:"WPI_RobotDriveDelayAndUpdateSafety.vi"("Delay (s)"=1.0, "RobotDriveDevRef"=w214) -> ("RobotDriveDevRef 2"=w215:T16)  [unwired: 8 in, 1 out]
          n117 = call-poly <vilib>:"WPI_RobotDriveArcadeDrive.vi"("Y axis value"=-0.25 ("X axis value"), "X axis value"=0.5, "RobotDriveDevRef"=w215) -> ("Motor Values"=w206:dbl[], "RobotDriveDevRef"=w216:T16)  [unwired: 1 in, 6 out]
          n118 = call <vilib>:"WPI_RobotDriveDelayAndUpdateSafety.vi"("Delay (s)"=0.5, "RobotDriveDevRef"=w216) -> ("RobotDriveDevRef 2"=w217:T16)  [unwired: 8 in, 1 out]
          n119 = call-poly <vilib>:"NT Write Value.vi"("Numeric Array"=w204, "Name"=w205) -> ()  [unwired: 9 in, 1 out]
          n120 = call-poly <vilib>:"NT Write Value.vi"("Numeric Array"=w206, "Name"=w205) -> ()  [unwired: 9 in, 1 out]
          n121 = call-poly <vilib>:"WPI_RobotDriveArcadeDrive.vi"("Y axis value"=0.0 ("X axis value"), "X axis value"=0.0, "RobotDriveDevRef"=w217) -> ("Motor Values"=w207:dbl[])  [unwired: 1 in, 7 out]
          n122 = call-poly <vilib>:"NT Write Value.vi"("Numeric Array"=w207, "Name"=w205) -> ()  [unwired: 9 in, 1 out]
        }
        frame Default {
          n123 = case shown="\"True\"" w222 {
            frame "False", Default {
            }
            frame "True" {
              w235 = FPGA_DIOChannel."DIO 1"  # B Channel
              w234 = FPGA_DIOChannel."DIO 0"  # A Channel
              w248 = FPGA_DIOChannel."DIO 1"  # B Channel
              w247 = FPGA_DIOChannel."DIO 0"  # A Channel
              w259 = FPGA_DIOChannel."DIO 1"  # B Channel
              w258 = FPGA_DIOChannel."DIO 0"  # A Channel
              w271 = FPGA_DIOChannel."DIO 1"  # B Channel
              w270 = FPGA_DIOChannel."DIO 0"  # A Channel
              w283 = FPGA_DIOChannel."DIO 1"  # B Channel
              w282 = FPGA_DIOChannel."DIO 0"  # A Channel
              w295 = FPGA_DIOChannel."DIO 1"  # B Channel
              w294 = FPGA_DIOChannel."DIO 0"  # A Channel
              w306 = FPGA_DIOChannel."DIO 1"  # B Channel
              w305 = FPGA_DIOChannel."DIO 0"  # A Channel
              (unwired) 0.0 ("Distance")
              # "in inches"
              # "in inches"
              # "in inches"
              # "in inches"
              # "in inches"
              # "in inches"
              # "in inches"
              n124 = call <vilib>:"WPI_DigitalInputOpen.vi"("DIO Channel"=w305) -> ("DigitalInputDevRef"=w302:T4)  [unwired: 1 in, 9 out]
              n125 = call <vilib>:"WPI_DigitalInputOpen.vi"("DIO Channel"=w306) -> ("DigitalInputDevRef"=w303:T4)  [unwired: 1 in, 9 out]
              n126 = call-poly <vilib>:"WPI_CounterToDigitalSource.vi"("DigitalInputDevRef"=w302) -> ("Digital Source"=w223:T5)  [unwired: 6 out]
              n127 = call-poly <vilib>:"WPI_CounterToDigitalSource.vi"("DigitalInputDevRef"=w303) -> ("Digital Source"=w304:T5)  [unwired: 6 out]
              n128 = call <vilib>:"WPI_EncoderOpen.vi"("DistancePerCount"=18.84955592153876, "BSource"=w304, "ASource"=w223) -> ("error out"=w299:errorcluster, "EncoderDevRef"=w300:T9)  [unwired: 5 in, 2 out]
              n129 = call <vilib>:"WPI_EncoderGet.vi"("error in (no error)"=w299, "EncoderDevRef"=w300) -> ("Distance"=w298:dbl)  [unwired: 4 in, 5 out]
              n130 = call <vilib>:"WPI_RobotDriveRefNum Registry Get.vi"("refnum name"="Left Right Motors") -> ("RobotDriveDevRef"=w325:T16)  [unwired: 9 in, 1 out]
              n131 = Equal?(x=w298, y=100.0) -> (x = y?=w296:bool)
              n132 = case shown="True" w296 {
                tunnel: w325 -> [w355 w359]
                tunnel: [w355 w356] -> w324
                frame False {
                }
                frame True {
                  n133 = call-poly <vilib>:"WPI_RobotDriveArcadeDrive.vi"("Y axis value"=0.05, "X axis value"=0.0, "RobotDriveDevRef"=w359) -> ("RobotDriveDevRef"=w356:T16)  [unwired: 6 in, 2 out]
                }
              }
              n134 = call <vilib>:"WPI_DigitalInputOpen.vi"("DIO Channel"=w294) -> ("DigitalInputDevRef"=w291:T4)  [unwired: 1 in, 9 out]
              n135 = call <vilib>:"WPI_DigitalInputOpen.vi"("DIO Channel"=w295) -> ("DigitalInputDevRef"=w292:T4)  [unwired: 1 in, 9 out]
              n136 = call-poly <vilib>:"WPI_CounterToDigitalSource.vi"("DigitalInputDevRef"=w291) -> ("Digital Source"=w290:T5)  [unwired: 6 out]
              n137 = call-poly <vilib>:"WPI_CounterToDigitalSource.vi"("DigitalInputDevRef"=w292) -> ("Digital Source"=w293:T5)  [unwired: 6 out]
              n138 = call <vilib>:"WPI_EncoderOpen.vi"("DistancePerCount"=18.84955592153876, "BSource"=w293, "ASource"=w290) -> ("error out"=w287:errorcluster, "EncoderDevRef"=w288:T9)  [unwired: 5 in, 2 out]
              n139 = call <vilib>:"WPI_EncoderGet.vi"("error in (no error)"=w287, "EncoderDevRef"=w288) -> ("Distance"=w286:dbl)  [unwired: 4 in, 5 out]
              n140 = call <vilib>:"WPI_RobotDriveDelayAndUpdateSafety.vi"("Delay (s)"=0.07, "RobotDriveDevRef"=w324) -> ("RobotDriveDevRef 2"=w320:T16)  [unwired: 8 in, 1 out]
              n141 = Equal?(x=w286, y=100.0) -> (x = y?=w284:bool)
              n142 = case shown="True" w284 {
                tunnel: w320 -> [w350 w354]
                tunnel: [w350 w351] -> w322
                frame False {
                }
                frame True {
                  n143 = call-poly <vilib>:"WPI_RobotDriveArcadeDrive.vi"("Y axis value"=0.15, "X axis value"=0.0, "RobotDriveDevRef"=w354) -> ("RobotDriveDevRef"=w351:T16)  [unwired: 6 in, 2 out]
                }
              }
              n144 = call <vilib>:"WPI_DigitalInputOpen.vi"("DIO Channel"=w282) -> ("DigitalInputDevRef"=w279:T4)  [unwired: 1 in, 9 out]
              n145 = call <vilib>:"WPI_DigitalInputOpen.vi"("DIO Channel"=w283) -> ("DigitalInputDevRef"=w280:T4)  [unwired: 1 in, 9 out]
              n146 = call-poly <vilib>:"WPI_CounterToDigitalSource.vi"("DigitalInputDevRef"=w279) -> ("Digital Source"=w278:T5)  [unwired: 6 out]
              n147 = call-poly <vilib>:"WPI_CounterToDigitalSource.vi"("DigitalInputDevRef"=w280) -> ("Digital Source"=w281:T5)  [unwired: 6 out]
              n148 = call <vilib>:"WPI_EncoderOpen.vi"("DistancePerCount"=18.84955592153876, "BSource"=w281, "ASource"=w278) -> ("error out"=w275:errorcluster, "EncoderDevRef"=w276:T9)  [unwired: 5 in, 2 out]
              n149 = call <vilib>:"WPI_EncoderGet.vi"("error in (no error)"=w275, "EncoderDevRef"=w276) -> ("Distance"=w274:dbl)  [unwired: 4 in, 5 out]
              n150 = call <vilib>:"WPI_RobotDriveDelayAndUpdateSafety.vi"("Delay (s)"=0.1, "RobotDriveDevRef"=w322) -> ("RobotDriveDevRef 2"=w317:T16)  [unwired: 8 in, 1 out]
              n151 = Equal?(x=w274, y=100.0) -> (x = y?=w272:bool)
              n152 = case shown="True" w272 {
                tunnel: w317 -> [w345 w349]
                tunnel: [w345 w346] -> w319
                frame False {
                }
                frame True {
                  n153 = call-poly <vilib>:"WPI_RobotDriveArcadeDrive.vi"("Y axis value"=0.3, "X axis value"=0.0, "RobotDriveDevRef"=w349) -> ("RobotDriveDevRef"=w346:T16)  [unwired: 6 in, 2 out]
                }
              }
              n154 = call <vilib>:"WPI_DigitalInputOpen.vi"("DIO Channel"=w270) -> ("DigitalInputDevRef"=w267:T4)  [unwired: 1 in, 9 out]
              n155 = call <vilib>:"WPI_DigitalInputOpen.vi"("DIO Channel"=w271) -> ("DigitalInputDevRef"=w268:T4)  [unwired: 1 in, 9 out]
              n156 = call-poly <vilib>:"WPI_CounterToDigitalSource.vi"("DigitalInputDevRef"=w267) -> ("Digital Source"=w266:T5)  [unwired: 6 out]
              n157 = call-poly <vilib>:"WPI_CounterToDigitalSource.vi"("DigitalInputDevRef"=w268) -> ("Digital Source"=w269:T5)  [unwired: 6 out]
              n158 = call <vilib>:"WPI_EncoderOpen.vi"("DistancePerCount"=18.84955592153876, "BSource"=w269, "ASource"=w266) -> ("error out"=w263:errorcluster, "EncoderDevRef"=w264:T9)  [unwired: 5 in, 2 out]
              n159 = call <vilib>:"WPI_EncoderGet.vi"("error in (no error)"=w263, "EncoderDevRef"=w264) -> ("Distance"=w262:dbl)  [unwired: 4 in, 5 out]
              n160 = call <vilib>:"WPI_RobotDriveDelayAndUpdateSafety.vi"("Delay (s)"=0.1, "RobotDriveDevRef"=w319) -> ("RobotDriveDevRef 2"=w315:T16)  [unwired: 8 in, 1 out]
              n161 = Equal?(x=w262, y=100.0) -> (x = y?=w260:bool)
              n162 = case shown="True" w260 {
                tunnel: w315 -> [w340 w344]
                tunnel: [w340 w341] -> w316
                frame False {
                }
                frame True {
                  n163 = call-poly <vilib>:"WPI_RobotDriveArcadeDrive.vi"("Y axis value"=0.5, "X axis value"=0.0, "RobotDriveDevRef"=w344) -> ("RobotDriveDevRef"=w341:T16)  [unwired: 6 in, 2 out]
                }
              }
              n164 = call <vilib>:"WPI_DigitalInputOpen.vi"("DIO Channel"=w258) -> ("DigitalInputDevRef"=w255:T4)  [unwired: 1 in, 9 out]
              n165 = call <vilib>:"WPI_DigitalInputOpen.vi"("DIO Channel"=w259) -> ("DigitalInputDevRef"=w256:T4)  [unwired: 1 in, 9 out]
              n166 = call-poly <vilib>:"WPI_CounterToDigitalSource.vi"("DigitalInputDevRef"=w255) -> ("Digital Source"=w254:T5)  [unwired: 6 out]
              n167 = call-poly <vilib>:"WPI_CounterToDigitalSource.vi"("DigitalInputDevRef"=w256) -> ("Digital Source"=w257:T5)  [unwired: 6 out]
              n168 = call <vilib>:"WPI_EncoderOpen.vi"("DistancePerCount"=18.84955592153876, "BSource"=w257, "ASource"=w254) -> ("error out"=w251:errorcluster, "EncoderDevRef"=w252:T9)  [unwired: 5 in, 2 out]
              n169 = call <vilib>:"WPI_EncoderGet.vi"("error in (no error)"=w251, "EncoderDevRef"=w252) -> ("Distance"=w250:dbl)  [unwired: 4 in, 5 out]
              n170 = call <vilib>:"WPI_RobotDriveDelayAndUpdateSafety.vi"("Delay (s)"=0.1, "RobotDriveDevRef"=w316) -> ("RobotDriveDevRef 2"=w311:T16)  [unwired: 8 in, 1 out]
              n171 = Equal?(x=w250, y=100.0) -> (x = y?=w237:bool)
              n172 = case shown="True" w237 {
                tunnel: w311 -> [w335 w339]
                tunnel: [w335 w336] -> w312
                frame False {
                }
                frame True {
                  n173 = call-poly <vilib>:"WPI_RobotDriveArcadeDrive.vi"("Y axis value"=0.7, "X axis value"=0.0, "RobotDriveDevRef"=w339) -> ("RobotDriveDevRef"=w336:T16)  [unwired: 6 in, 2 out]
                }
              }
              n174 = call <vilib>:"WPI_DigitalInputOpen.vi"("DIO Channel"=w247) -> ("DigitalInputDevRef"=w244:T4)  [unwired: 1 in, 9 out]
              n175 = call <vilib>:"WPI_DigitalInputOpen.vi"("DIO Channel"=w248) -> ("DigitalInputDevRef"=w245:T4)  [unwired: 1 in, 9 out]
              n176 = call-poly <vilib>:"WPI_CounterToDigitalSource.vi"("DigitalInputDevRef"=w244) -> ("Digital Source"=w243:T5)  [unwired: 6 out]
              n177 = call-poly <vilib>:"WPI_CounterToDigitalSource.vi"("DigitalInputDevRef"=w245) -> ("Digital Source"=w246:T5)  [unwired: 6 out]
              n178 = call <vilib>:"WPI_EncoderOpen.vi"("DistancePerCount"=18.84955592153876, "BSource"=w246, "ASource"=w243) -> ("error out"=w240:errorcluster, "EncoderDevRef"=w241:T9)  [unwired: 5 in, 2 out]
              n179 = call <vilib>:"WPI_EncoderGet.vi"("error in (no error)"=w240, "EncoderDevRef"=w241) -> ("Distance"=w239:dbl)  [unwired: 4 in, 5 out]
              n180 = call <vilib>:"WPI_RobotDriveDelayAndUpdateSafety.vi"("Delay (s)"=0.1, "RobotDriveDevRef"=w312) -> ("RobotDriveDevRef 2"=w308:T16)  [unwired: 8 in, 1 out]
              n181 = Equal?(x=w239, y=100.0) -> (x = y?=w236:bool)
              n182 = case shown="True" w236 {
                tunnel: w308 -> [w330 w334]
                tunnel: [w330 w331] -> w309
                frame False {
                }
                frame True {
                  n183 = call-poly <vilib>:"WPI_RobotDriveArcadeDrive.vi"("Y axis value"=0.9, "X axis value"=0.0, "RobotDriveDevRef"=w334) -> ("RobotDriveDevRef"=w331:T16)  [unwired: 6 in, 2 out]
                }
              }
              n184 = call <vilib>:"WPI_DigitalInputOpen.vi"("DIO Channel"=w234) -> ("DigitalInputDevRef"=w231:T4)  [unwired: 1 in, 9 out]
              n185 = call <vilib>:"WPI_DigitalInputOpen.vi"("DIO Channel"=w235) -> ("DigitalInputDevRef"=w232:T4)  [unwired: 1 in, 9 out]
              n186 = call-poly <vilib>:"WPI_CounterToDigitalSource.vi"("DigitalInputDevRef"=w231) -> ("Digital Source"=w230:T5)  [unwired: 6 out]
              n187 = call-poly <vilib>:"WPI_CounterToDigitalSource.vi"("DigitalInputDevRef"=w232) -> ("Digital Source"=w233:T5)  [unwired: 6 out]
              n188 = call <vilib>:"WPI_EncoderOpen.vi"("DistancePerCount"=18.84955592153876, "BSource"=w233, "ASource"=w230) -> ("error out"=w227:errorcluster, "EncoderDevRef"=w228:T9)  [unwired: 5 in, 2 out]
              n189 = call <vilib>:"WPI_EncoderGet.vi"("error in (no error)"=w227, "EncoderDevRef"=w228) -> ("Distance"=w226:dbl)  [unwired: 4 in, 5 out]
              n190 = call <vilib>:"WPI_RobotDriveDelayAndUpdateSafety.vi"("Delay (s)"=0.1, "RobotDriveDevRef"=w309) -> ("RobotDriveDevRef 2"=w307:T16)  [unwired: 8 in, 1 out]
              n191 = Equal?(x=w226, y=100.0) -> (x = y?=w224:bool)
              n192 = case shown="True" w224 {
                tunnel: w307 -> [_ w329]
                frame False {
                }
                frame True {
                  n193 = call-poly <vilib>:"WPI_RobotDriveArcadeDrive.vi"("Y axis value"=0.5, "X axis value"=0.0, "RobotDriveDevRef"=w329) -> ()  [unwired: 6 in, 3 out]
                }
              }
            }
          }
        }
      }
    }
    frame Enabled {
    }
  }
  n194 = Index Array(array=w3, index #1=2 ("index")) -> ()  [unwired: 1 in, 2 out]
  n195 = call-poly <vilib>:"NT Write Value.vi"("Numeric Array"=w3, "Name"="Joystick 0/Axes") -> ()  [unwired: 9 in, 1 out]
